vi "close.vi"(8 "error in":errorcluster, 11 "module in":refnum<class "E2E Runtime (UDP).lvclass">) -> (0 "error out":errorcluster)   [LabVIEW 2015, in "E2E Runtime (UDP).lvclass"]
doc: "Provides an interface for terminating a module instance. While this interface performs no operations, a child should close and deallocate any open references or memory."
uses:
  E2E Runtime (UDP).lvclass
  E2E Runtime (UDP).lvclass/E2E Runtime (UDP).ctl
  <vilib>/NI/Tag Bus Module Framework/runtime/TBM module execution interface.lvclass
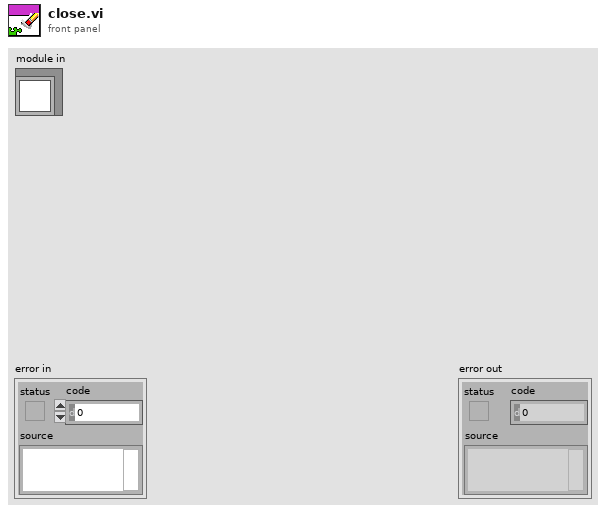
[diagram p1: front panel]
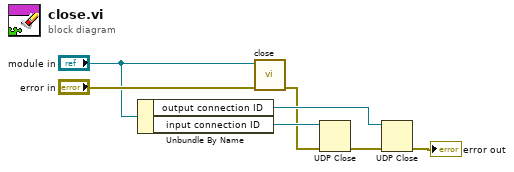
[diagram p0: block diagram]
diagram:
  n1 = Unbundle By Name("module in") -> ("output connection ID"=w4:refnum<k16>, "input connection ID"=w5:refnum<k16>)
  n2 = call-parent "close.vi"("error in"="error in", "module in"="module in") -> ("error out"=w1:errorcluster)  [unwired: 9 in]
  n3 = UDP Close(connection ID=w5, 8:w1) -> (error out=w3:errorcluster)  [unwired: 1 out]
  n4 = UDP Close(connection ID=w4, 8:w3) -> (error out=→"error out":errorcluster)  [unwired: 1 out]
